vi "Open.vi"(8 "error in (no error)":errorcluster, 11 "Test Case in":refnum<class "Test Case.lvclass">) -> (0 "error out":errorcluster, 3 "Test Case out":refnum<class "Test Case.lvclass">)   [LabVIEW 2017, in "Test Case.lvclass"]
doc: "Opens the document associated with the test case."
uses:
  Test Case.lvclass
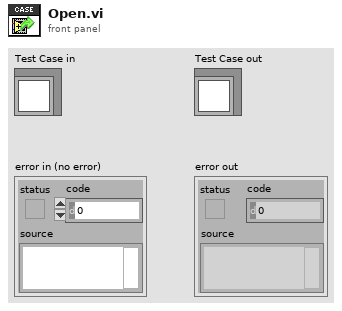
[diagram p1: front panel]
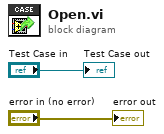
[diagram p0: block diagram]
diagram:
  "error out" <- "error in (no error)"
  "Test Case out" <- "Test Case in"
